vi "Write multi coils.vi"(2 "error in":errorcluster, 3 "coils to write":bool[](array[boolean]), 4 "starting address":u16) -> (0 "error IO":errorcluster, 1 "State":bool)   [LabVIEW 2022 SP3]
uses:
  <vilib>/NI/Modbus Library/API/Master/Modbus Master.lvclass
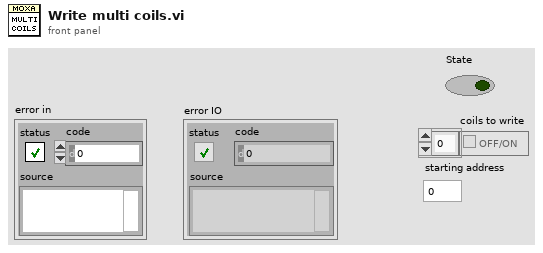
[diagram p1: front panel]
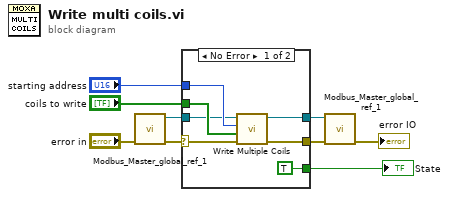
[diagram p0: block diagram]
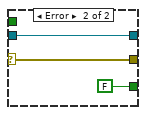
[diagram p2: hidden frame]
diagram:
  n1 = call "Modbus_Master_global_ref_1.vi"("error in (no error) 2"="error in") -> ("error out 2"=w4:errorcluster, "Modbus Master out"=w6:refnum<class "Modbus Master.lvclass">)  [unwired: 9 in]
  n2 = case shown="No Error" w4 {
    selector: w4 -> [w11 w19]
    tunnel: "coils to write" -> [w13 _]
    tunnel: "starting address" -> [w14 _]
    tunnel: [w16 w19] -> w3
    tunnel: [TRUE FALSE] -> w7
    tunnel: w6 -> [w12 w17]
    tunnel: [w10 w17] -> w1
    frame No Error {
      n3 = call-dynamic "Write Multiple Coils.vi"("error in"=w11, "coils to write"=w13, "starting address"=w14, "Modbus master in"=w12) -> ("error out"=w16:errorcluster, "Modbus master out"=w10:refnum<class "Modbus Master.lvclass">)  [unwired: 6 in]
    }
    frame Error {
    }
  }
  "State" <- w7
  n4 = call "Modbus_Master_global_ref_1.vi"("error in (no error) 2"=w3, "Modbus Master In"=w1) -> ("error out 2"=→"error IO":errorcluster)  [unwired: 8 in, 1 out]
